vi "AC_CloseDriver.vi"(1 "hDevice(in)":u32) -> (0 "hDevice(out)":u32)   [LabVIEW 2015]
uses:
  acpci.dll
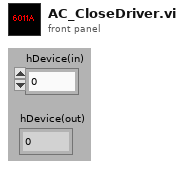
[diagram p1: front panel]
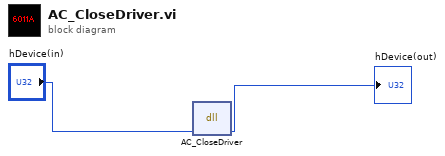
[diagram p0: block diagram]
diagram:
  n1 = dll-call lib="PTH2|abs F2.技术库labviewVI小程序:基于Labview的直流伺服电机位置控制系统设计\t源程序\tACPCI.DLL" fn="AC_CloseDriver"("hDevice"="hDevice(in)") -> ("hDevice"=→"hDevice(out)":u32)  [unwired: 4 in, 2 out]
